vi "Get Additional data.vi"(11 "Additional Data":variant) -> (3 "Formated Additional data":string)   [LabVIEW 2023]
doc: "Converting data from Variant to defined data types and converting them to Formated string.\nPossible formats CAN message, Number, Array of numbers, String"
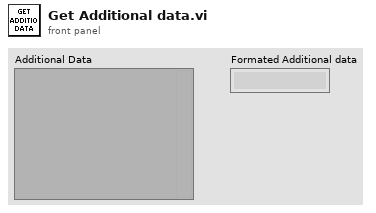
[diagram p1: front panel]
types:
  T1 = cluster{"ID":u32, "MSGTYPE":u8, "LEN":u8, "DATA[0]":u8, "DATA[1]":u8, "DATA[2]":u8, "DATA[3]":u8, "DATA[4]":u8, "DATA[5]":u8, "DATA[6]":u8, "DATA[7]":u8}
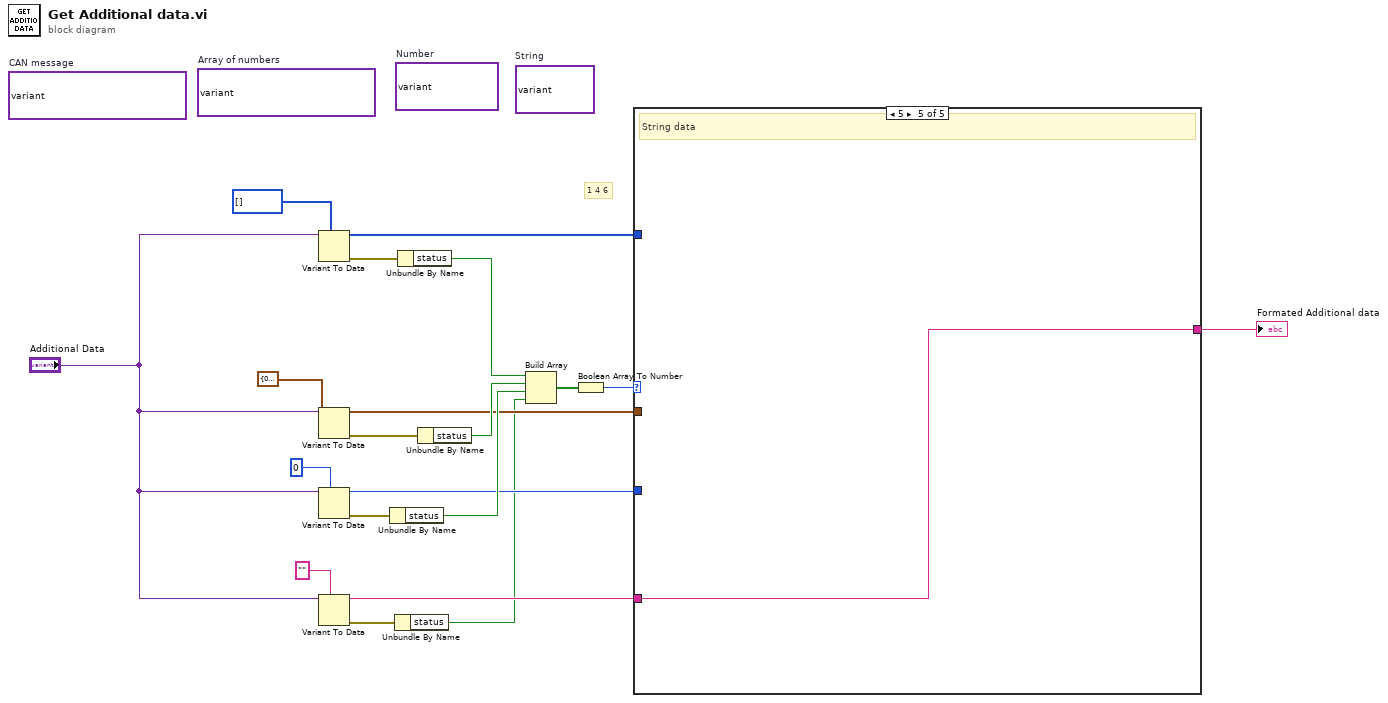
[diagram p0: block diagram]
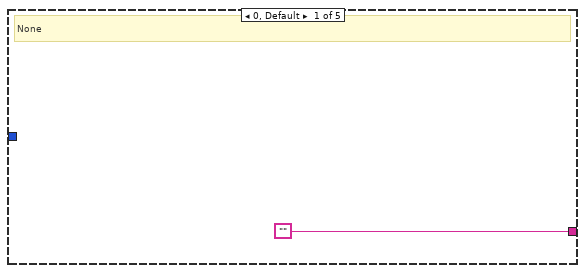
[diagram p2: hidden frame]
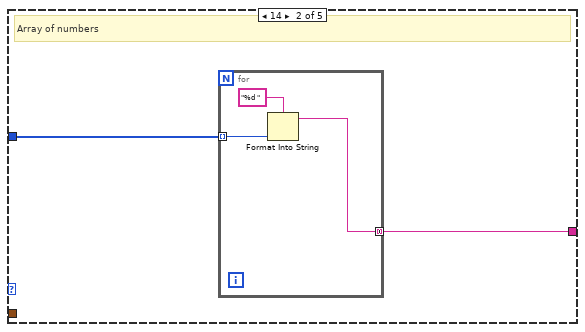
[diagram p3: hidden frame]
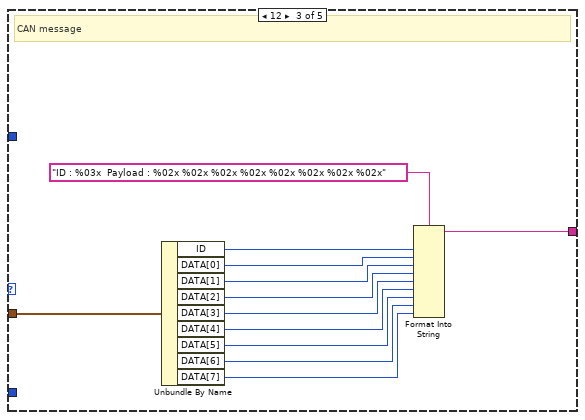
[diagram p4: hidden frame]
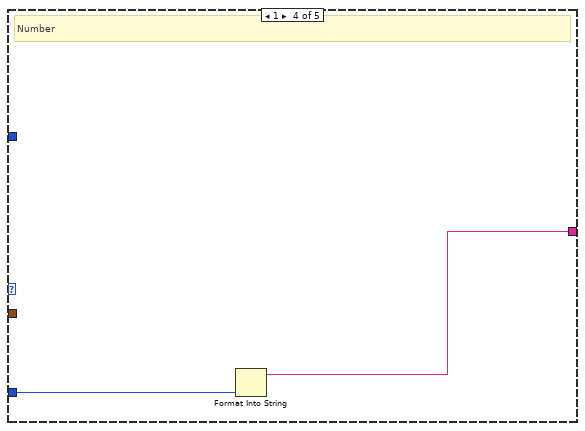
[diagram p5: hidden frame]
diagram:
  (unwired) variant  # String
  (unwired) variant  # Number
  (unwired) variant  # Array of numbers
  (unwired) variant  # CAN message
  # "1 4 6"
  n1 = Variant To Data(type=i32[] [], Variant="Additional Data") -> (data=w7:i32[], error out=w17:errorcluster)  [unwired: 1 in]
  n2 = Variant To Data(type=T1 {"ID"=0, "MSGTYPE"=0, "LEN"=0, "DATA[0]"=0, "DATA[1]"=0, "DATA[2]"=0, "DATA[3]"=0, "DATA[4]"=0, "DATA[5]"=0, "DATA[6]"=0, "DATA[7]"=0} ("MessageBuffer out"), Variant="Additional Data") -> (data=w8:T1, error out=w16:errorcluster)  [unwired: 1 in]
  n3 = Variant To Data(type=0, Variant="Additional Data") -> (data=w9:i32, error out=w15:errorcluster)  [unwired: 1 in]
  n4 = Variant To Data(type="", Variant="Additional Data") -> (data=w3:string, error out=w5:errorcluster)  [unwired: 1 in]
  n5 = Unbundle By Name(w15) -> ("status"=w12:bool)
  n6 = Unbundle By Name(w5) -> ("status"=w2:bool)
  n7 = Unbundle By Name(w17) -> ("status"=w14:bool)
  n8 = Unbundle By Name(w16) -> ("status"=w13:bool)
  n9 = Build Array(w14, w13, w12, w2) -> (w11:bool[])
  n10 = Boolean Array To Number(Boolean array=w11) -> (number=w10:u32)
  n11 = case shown="5" w10 {
    tunnel: w9 -> [_ _ _ w40 _]
    tunnel: w8 -> [_ _ w27 _ _]
    tunnel: w7 -> [_ w23 _ _ _]
    tunnel: ["" w22 w28 w39 w41] -> w6
    tunnel: w3 -> [_ _ _ _ w41]
    frame 0, Default {
      # "None"
    }
    frame 14 {
      # "Array of numbers"
      n12 = for {
        tunnel: w23 -> [w26] mode=indexing
        tunnel: [w24] -> w22 mode=concatenating
        n13 = Format Into String(format string="%d ", w26) -> (resulting string=w24:string)  [unwired: 2 in, 1 out]
      }
    }
    frame 12 {
      # "CAN message"
      n14 = Unbundle By Name(w27) -> ("ID"=w37:u32, "DATA[0]"=w36:u8, "DATA[1]"=w35:u8, "DATA[2]"=w34:u8, "DATA[3]"=w33:u8, "DATA[4]"=w32:u8, "DATA[5]"=w31:u8, "DATA[6]"=w30:u8, "DATA[7]"=w29:u8)
      n15 = Format Into String(format string="ID : %03x  Payload : %02x %02x %02x %02x %02x %02x %02x %02x", w37, w36, w35, w34, w33, w32, w31, w30, w29) -> (resulting string=w28:string)  [unwired: 2 in, 1 out]
    }
    frame 1 {
      # "Number"
      n16 = Format Into String(w40) -> (resulting string=w39:string)  [unwired: 3 in, 1 out]
    }
    frame 5 {
      # "String data"
    }
  }
  "Formated Additional data" <- w6
